vi "Error.vi"(8 "error in (no error)":errorcluster, 10 "Data":variant) -> (0 "error out":errorcluster)   [LabVIEW 2023, in "Template.lvlib"]
doc: "VI used to call ERROR in the Message Handling Loop"
uses:
  Type Def/Message Data.ctl
  Template.lvlib
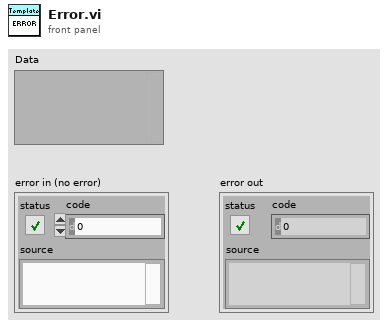
[diagram p1: front panel]
types:
  T1 = typedef "Template.lvlib/Message Data.ctl" = cluster{"Message":string, "Data":variant}
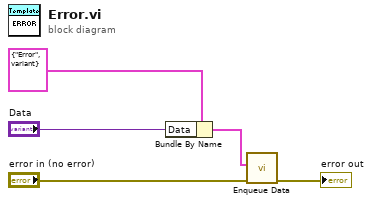
[diagram p0: block diagram]
diagram:
  n1 = Bundle By Name(cluster=T1 {"Message"="Error", "Data"=variant} ("Message Data"), "Data"="Data") -> (w2:T1)
  n2 = call "Enqueue Data.vi"("error in (no error)"="error in (no error)", "Message Data"=w2) -> ("error out"=→"error out":errorcluster)  [unwired: 9 in]
